vi "Host - Get Masters.vi"(8 "error in (no error)":errorcluster, 11 "All ECAT Masters":refnum<k21>[](array[refnum])) -> (0 "error out":errorcluster, 3 "Array":T1[](array[typedef]))   [LabVIEW 2015, in "Scan Engine Custom Device.lvlib"]
uses:
  Scan Engine Custom Device.lvlib
  Type Defs/Host - Master.ctl
  Type Defs/Host - Slave.ctl
  Type Defs/Host - Module.ctl
  <resource>/objmgr/IndComECAT.rc
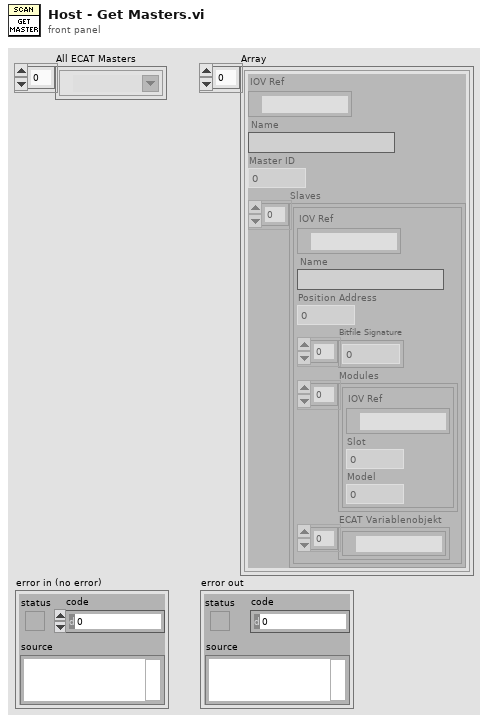
[diagram p1: front panel]
types:
  T1 = typedef "Scan Engine Custom Device.lvlib/Host - Master.ctl" = cluster{"IOV Ref":refnum<k21>, "Name":string, "Master ID":u32, "Slaves":T2[]}
  T2 = typedef "Scan Engine Custom Device.lvlib/Host - Slave.ctl" = cluster{"IOV Ref":refnum<k21>, "Name":string, "Position Address":u16, "Bitfile Signature":u8[], "Modules":T3[], "ECAT Variablenobjekt":refnum<k21>[]}
  T3 = typedef "Scan Engine Custom Device.lvlib/Host - Module.ctl" = cluster{"IOV Ref":refnum<k21>, "Slot":u32, "Model":u32}
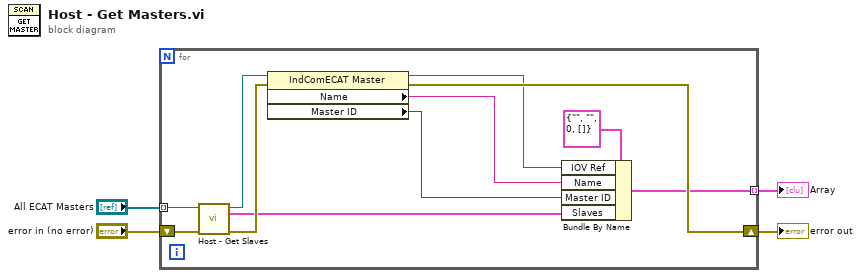
[diagram p0: block diagram]
diagram:
  n1 = for {
    tunnel: "All ECAT Masters" -> [w15] mode=indexing
    tunnel: [w5] -> w4 mode=indexing
    shift-right: [w11] -> w3
    shift-left: "error in (no error)" -> [w14]
    n2 = call "Host - Get Slaves.vi"("error in (no error)"=w14, "Master Ref in"=w15) -> ("error out"=w12:errorcluster, "Slaves"=w6:T2[], "Master Ref out"=w13:refnum<k21>)  [unwired: 7 in]
    n3 = property class="IndComECAT Master"(reference=w13, error in=w12) -> (reference out=w9:refnum<k21>, error out=w11:errorcluster, "Name"=w8:string, "Master ID"=w7:u32)
    n4 = Bundle By Name(cluster=T1 {"IOV Ref"="", "Name"="", "Master ID"=0, "Slaves"=[]} ("Master"), "IOV Ref"=w9, "Name"=w8, "Master ID"=w7, "Slaves"=w6) -> (w5:T1)
  }
  "Array" <- w4
  "error out" <- w3
